vi "setILCPort.vi"(10 "ILC Port":refnum<visa-resource-name>, 11 "DesktopModbus in":refnum<class "DesktopModbus.lvclass">) -> (3 "DesktopModbus out":refnum<class "DesktopModbus.lvclass">)   [LabVIEW 2015, in "DesktopModbus.lvclass"]
uses:
  DesktopModbus.lvclass
  DesktopModbus.lvclass/DesktopModbus.ctl
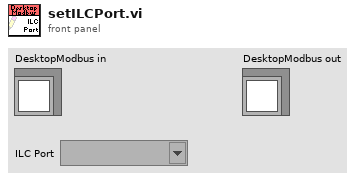
[diagram p1: front panel]
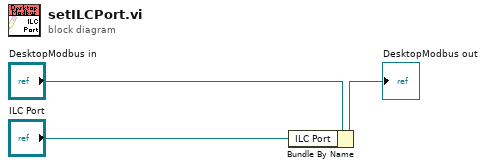
[diagram p0: block diagram]
diagram:
  n1 = Bundle By Name(cluster="DesktopModbus in", "ILC Port"="ILC Port") -> (→"DesktopModbus out":refnum<class "DesktopModbus.lvclass">)
